vi "Convert�mToPixels.vi"(8 "error in (no error)":errorcluster, 10 "Parameters":T1={"number of planes"=4, "z step"=1.9999999999999998e-05, "pixel dwell time"=1.0000000000000001e-11, "z frequency"=10.0, "number of pixels"=100, "smooth points"=10, "smooth line"=10, "Sine\nSawtooth"=FALSE, "PointSorting"=0, "Sort Points"=FALSE, "X-pixels"=256.0, "Y-lines"=256.0, "pixelstoµm"=256.0, "zoom"=1.0, "Time offset"=1.0000000000000001e-11} {"zoom" min=0.5 step=0.1; "Y-lines" min=1 step=1; "X-pixels" min=1 step=1; "PointSorting" items=["No Difference", "Every Second Point", "Down / Up"]; "smooth line" min=1; "smooth points" min=1; "number of pixels" min=1; "z frequency" format="%_4g"; "number of planes" min=1}, 11 "Point coordinates (um)":dbl[][](array[numeric])) -> (0 "error out":errorcluster, 3 "Point coordinates (pixels)":dbl[][](array[numeric]))   [LabVIEW 2010]
uses:
  TypeDefs/ParameterCluster.ctl
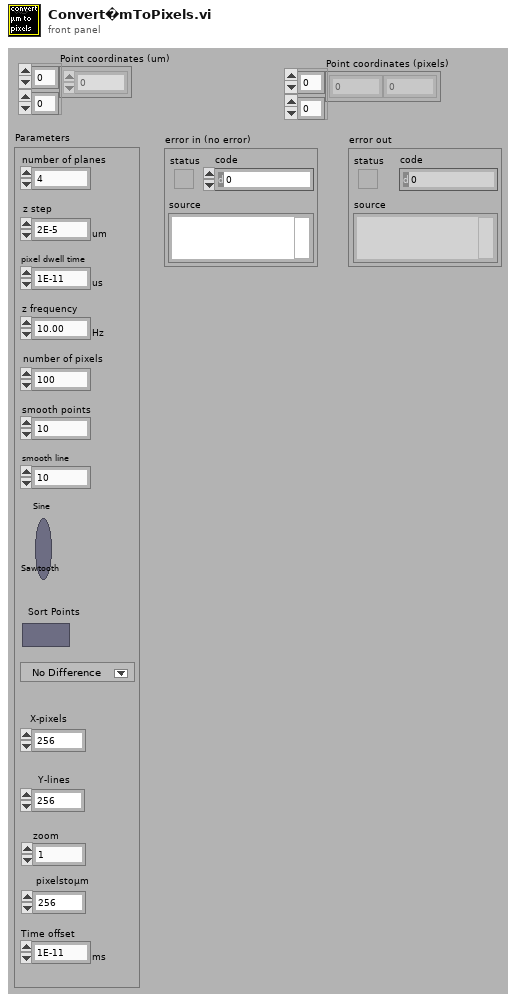
[diagram p1: front panel]
types:
  T1 = typedef "ParameterCluster.ctl" = cluster{"number of planes":i32, "z step":dbl[unit], "pixel dwell time":dbl[unit], "z frequency":dbl[unit], "number of pixels":i32, "smooth points":i32, "smooth line":i32, "Sine\nSawtooth":bool, "PointSorting":u16, "Sort Points":bool, "X-pixels":sgl, "Y-lines":sgl, "pixelstoµm":dbl, "zoom":dbl, "Time offset":dbl[unit]}
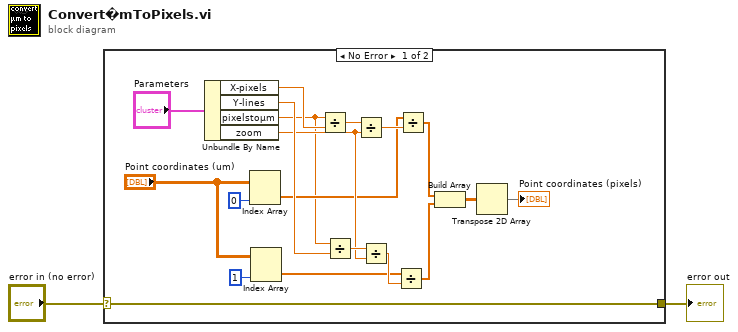
[diagram p0: block diagram]
diagram:
  n1 = case shown="No Error" "error in (no error)" {
    selector: "error in (no error)" -> [w17 w22]
    tunnel: [w17 w22] -> w1
    frame No Error {
      n2 = Unbundle By Name("Parameters") -> ("X-pixels"=w10:sgl, "Y-lines"=w9:sgl, "pixelstoµm"=w4:dbl, "zoom"=w8:dbl)
      n3 = Index Array(array="Point coordinates (um)", index (col)=0 ("disabled index (col)")) -> (element=w7:dbl[])  [unwired: 1 in]
      n4 = Index Array(array="Point coordinates (um)", index (col)=1 ("disabled index (col)")) -> (element=w6:dbl[])  [unwired: 1 in]
      n5 = Divide(x=w4, y=w10) -> (x/y=w11:dbl)
      n6 = Divide(x=w4, y=w9) -> (x/y=w12:dbl)
      n7 = Divide(x=w11, y=w8) -> (x/y=w13:dbl)
      n8 = Divide(x=w12, y=w8) -> (x/y=w15:dbl)
      n9 = Divide(x=w6, y=w15) -> (x/y=w16:dbl[])
      n10 = Divide(x=w7, y=w13) -> (x/y=w14:dbl[])
      n11 = Build Array(w14, w16) -> (w5:dbl[][])
      n12 = Transpose 2D Array(2D array=w5) -> (transposed array=→"Point coordinates (pixels)":dbl[][])
    }
    frame Error {
    }
  }
  "error out" <- w1
